vi "Relay Control.vi"(0 "RFCalAndFixtureCharact.Common.lvlib:Path.lvclass":refnum<class "Path.lvclass">, 5 "TSM Context":T1, 11 "error in":errorcluster) -> (15 "error out":errorcluster)   [LabVIEW 2023]
uses:
  Common/Base Classes/Path/Path.lvclass
  <vilib>/NI_TestStand_SemiconductorModule/NI_TestStand_Semiconductor_Module.lvlibp/PinMap/General/SemiconductorModuleContext.ctl
  38b3e3b7-67cf-4d14-9388-074a1d97d46a.vi
  <vilib>/NI_TestStand_SemiconductorModule/NI_TestStand_Semiconductor_Module.lvlibp/PinMap/Relay Driver/ApplyRelayConfiguration.vi
  <vilib>/Comparison/Equal/Equal Functor/Equal Functor.lvclass
  <vilib>/NI_TestStand_SemiconductorModule/NI_TestStand_Semiconductor_Module.lvlibp
  Common/RFCalAndFixtureCharact.Common.lvlib
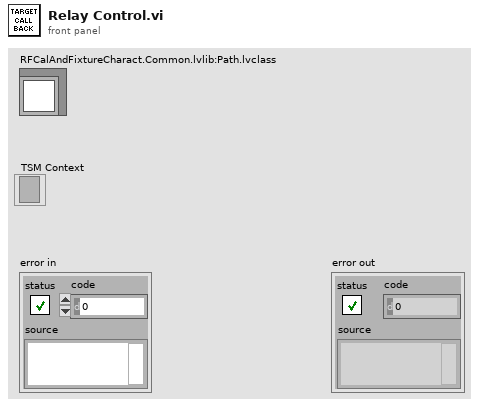
[diagram p1: front panel]
types:
  T1 = typedef "NI_TestStand_Semiconductor_Module.lvlibp/SemiconductorModuleContext.ctl" = refnum<k7>
  T2 = typedef "Path Types.ctl" = enum16{"SG Path", "SA Path", "Vector Path"}
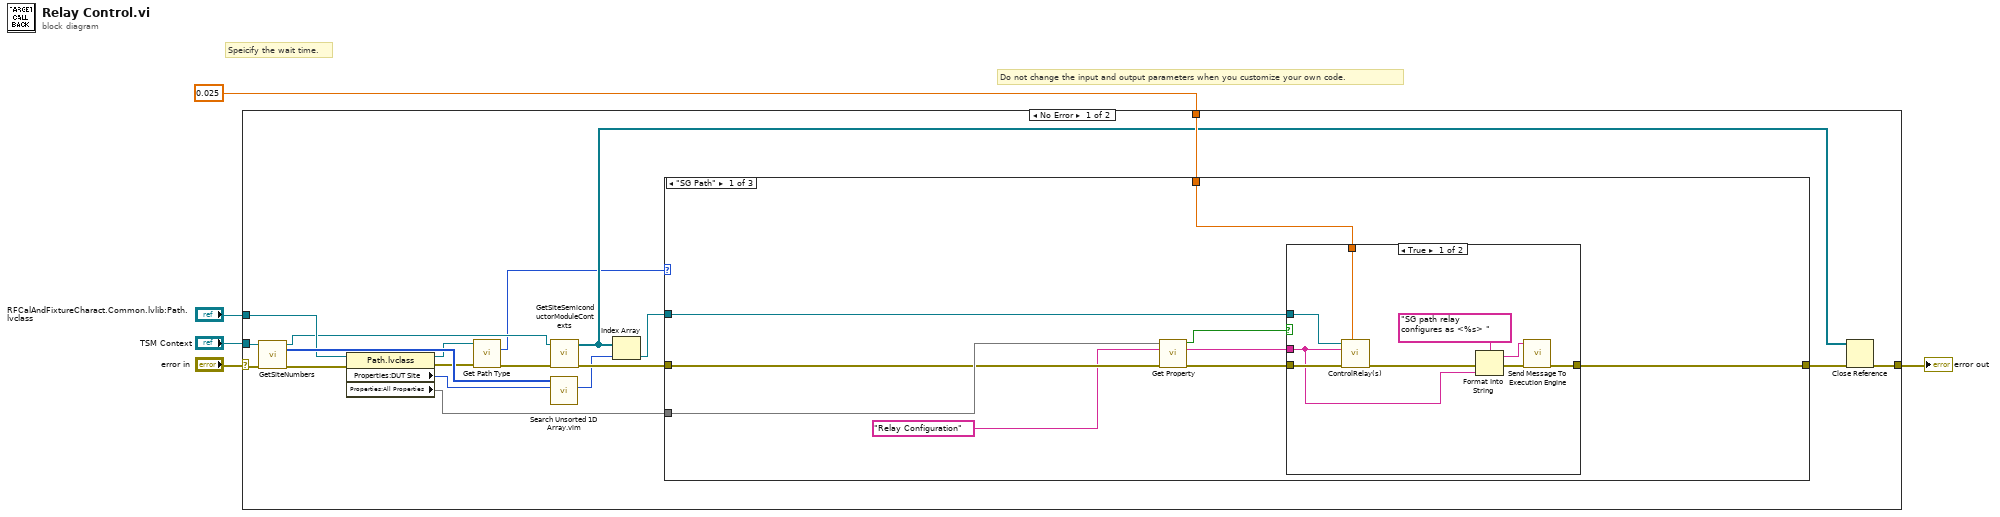
[diagram p0: block diagram]
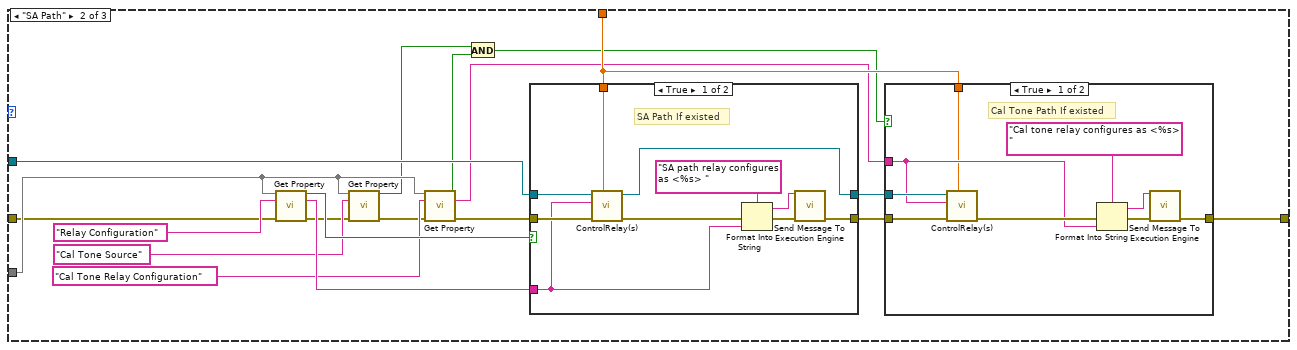
[diagram p3: hidden frame]
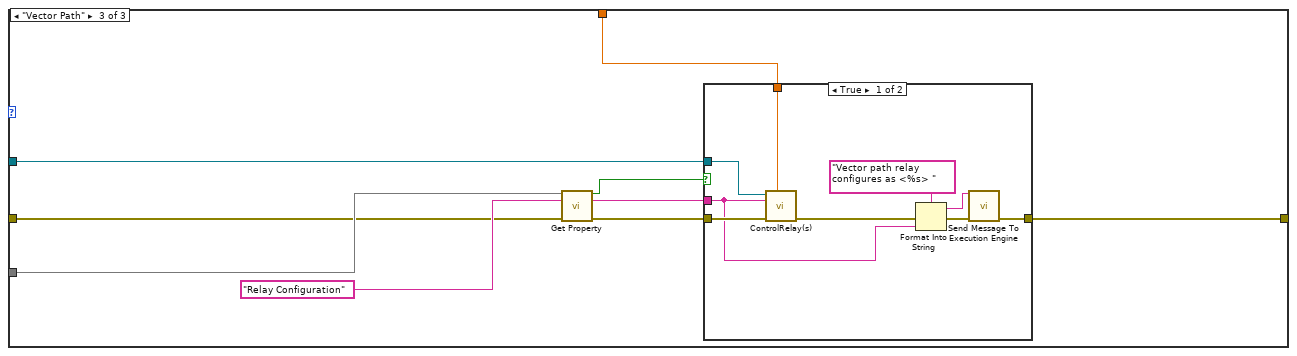
[diagram p6: hidden frame]
diagram:
  # "Speicify the wait time."
  # "Do not change the input and output parameters when you customize your own code."
  n1 = case shown="No Error" "error in" {
    selector: "error in" -> [w12 w104]
    tunnel: "RFCalAndFixtureCharact.Common.lvlib:Path.lvclass" -> [w11 _]
    tunnel: [w17 w104] -> w3
    tunnel: "TSM Context" -> [w24 _]
    tunnel: 0.025 ("Wait (s)") -> [w15 _]
    frame No Error {
      n2 = call <vilib>:"GetSiteNumbers.vi"("error in (no error)"=w12, "Semiconductor Module Context"=w24) -> ("error out"=w14:errorcluster, "Site Numbers"=w23:i32[], "Semiconductor Module Context Out"=w8:T1)  [unwired: 6 in, 1 out]
      n3 = property class="Path.lvclass"(reference=w11, error in=w14) -> (reference out=w9:refnum<class "Path.lvclass">, error out=w10:errorcluster, "Properties:DUT Site"=w21:i32, "Properties:All Properties"=w16:map{string, string})
      n4 = call "Get Path Type.vi"("Path in"=w9, "error in"=w10) -> ("Path Type"=w6:T2, "error out"=w7:errorcluster)  [unwired: 11 in, 1 out]
      n5 = call "Search Unsorted 1D Array.vim"("element"=w21, "unsorted 1D array"=w23) -> ("index of element"=w20:i32)  [unwired: 9 in]
      n6 = call <vilib>:"GetSiteSemiconductorModuleContexts.vi"("error in (no error)"=w7, "Semiconductor Module Context"=w8) -> ("error out"=w22:errorcluster, "Site Semiconductor Module Contexts"=w13:T1[])  [unwired: 8 in]
      n7 = Index Array(array=w13, index=w20) -> (element=w19:T1)
      n8 = case shown="\"SG Path\"" w6 {
        tunnel: w22 -> [w27 w50 w86]
        tunnel: w19 -> [w33 w62 w93]
        tunnel: [w31 w44 w91] -> w18
        tunnel: w16 -> [w30 w53 w90]
        tunnel: w15 -> [w32 w59 w92]
        frame "SG Path" {
          # "SG Path"
          n9 = call "Get Property.vi"("Properties"=w30, "Property Name"="Relay Configuration", "error in"=w27) -> ("Non-empty Value Found"=w29:bool, "Value"=w28:string, "error out"=w26:errorcluster)  [unwired: 10 in]
          n10 = case shown="True" w29 {
            tunnel: w28 -> [w35 _]
            tunnel: w26 -> [w38 w43]
            tunnel: [w39 w43] -> w31
            tunnel: w33 -> [w36 _]
            tunnel: w32 -> [w34 _]
            frame True {
              n11 = call-poly <vilib>:"ControlRelay(s).vi"("Wait (s)"=w34, "error in (no error)"=w38, "Relay Configuration"=w35, "Semiconductor Module Context"=w36) -> ("error out"=w37:errorcluster)  [unwired: 6 in, 1 out]
              n12 = Format Into String(format string="SG path relay configures as <%s> ", error in=w37, w35) -> (resulting string=w40:string, error out=w42:errorcluster)  [unwired: 1 in]
              n13 = call "Send Message To Execution Engine.vi"("Message"=w40, "error in (no error)"=w42) -> ("error out"=w39:errorcluster)  [unwired: 13 in]
            }
            frame False {
            }
          }
        }
        frame "SA Path" {
          # "SA Path"
          n14 = call "Get Property.vi"("Properties"=w53, "Property Name"="Relay Configuration", "error in"=w50) -> ("Non-empty Value Found"=w57:bool, "Value"=w56:string, "error out"=w49:errorcluster)  [unwired: 10 in]
          n15 = call "Get Property.vi"("Properties"=w53, "Property Name"="Cal Tone Source", "error in"=w49) -> ("Non-empty Value Found"=w45:bool, "error out"=w48:errorcluster)  [unwired: 10 in, 1 out]
          n16 = call "Get Property.vi"("Properties"=w53, "Property Name"="Cal Tone Relay Configuration", "error in"=w48) -> ("Non-empty Value Found"=w46:bool, "Value"=w51:string, "error out"=w47:errorcluster)  [unwired: 10 in]
          n17 = And(x=w45, y=w46) -> (x .and. y?=w52:bool)
          n18 = case shown="True" w57 {
            tunnel: w56 -> [w75 _]
            tunnel: w47 -> [w78 w84]
            tunnel: [w79 w84] -> w61
            tunnel: w62 -> [w76 w83]
            tunnel: w59 -> [w74 _]
            tunnel: [w73 w83] -> w60
            frame True {
              # "SA Path If existed"
              n19 = call-poly <vilib>:"ControlRelay(s).vi"("Wait (s)"=w74, "error in (no error)"=w78, "Relay Configuration"=w75, "Semiconductor Module Context"=w76) -> ("error out"=w77:errorcluster, "Semiconductor Module Context Out"=w73:T1)  [unwired: 6 in]
              n20 = Format Into String(format string="SA path relay configures as <%s> ", error in=w77, w75) -> (resulting string=w80:string, error out=w82:errorcluster)  [unwired: 1 in]
              n21 = call "Send Message To Execution Engine.vi"("Message"=w80, "error in (no error)"=w82) -> ("error out"=w79:errorcluster)  [unwired: 13 in]
            }
            frame False {
            }
          }
          n22 = case shown="True" w52 {
            tunnel: w51 -> [w64 _]
            tunnel: w61 -> [w67 w72]
            tunnel: [w68 w72] -> w44
            tunnel: w60 -> [w65 _]
            tunnel: w59 -> [w63 _]
            frame True {
              # "Cal Tone Path If existed"
              n23 = call-poly <vilib>:"ControlRelay(s).vi"("Wait (s)"=w63, "error in (no error)"=w67, "Relay Configuration"=w64, "Semiconductor Module Context"=w65) -> ("error out"=w66:errorcluster)  [unwired: 6 in, 1 out]
              n24 = Format Into String(format string="Cal tone relay configures as <%s> ", error in=w66, w64) -> (resulting string=w69:string, error out=w71:errorcluster)  [unwired: 1 in]
              n25 = call "Send Message To Execution Engine.vi"("Message"=w69, "error in (no error)"=w71) -> ("error out"=w68:errorcluster)  [unwired: 13 in]
            }
            frame False {
            }
          }
        }
        frame "Vector Path" {
          # "Vector Path"
          n26 = call "Get Property.vi"("Properties"=w90, "Property Name"="Relay Configuration", "error in"=w86) -> ("Non-empty Value Found"=w88:bool, "Value"=w87:string, "error out"=w85:errorcluster)  [unwired: 10 in]
          n27 = case shown="True" w88 {
            tunnel: w87 -> [w95 _]
            tunnel: w85 -> [w98 w103]
            tunnel: [w99 w103] -> w91
            tunnel: w93 -> [w96 _]
            tunnel: w92 -> [w94 _]
            frame True {
              n28 = call-poly <vilib>:"ControlRelay(s).vi"("Wait (s)"=w94, "error in (no error)"=w98, "Relay Configuration"=w95, "Semiconductor Module Context"=w96) -> ("error out"=w97:errorcluster)  [unwired: 6 in, 1 out]
              n29 = Format Into String(format string="Vector path relay configures as <%s> ", error in=w97, w95) -> (resulting string=w100:string, error out=w102:errorcluster)  [unwired: 1 in]
              n30 = call "Send Message To Execution Engine.vi"("Message"=w100, "error in (no error)"=w102) -> ("error out"=w99:errorcluster)  [unwired: 13 in]
            }
            frame False {
            }
          }
        }
      }
      n31 = Close Reference(reference=w13, error in (no error)=w18) -> (error out=w17:errorcluster)
    }
    frame Error {
    }
  }
  "error out" <- w3
